vi "PPL RT Driver VI_InlineAsync.vi"(7 "Operation":T1, 11 "Device Reference in":T2 format="%.0x") -> (0 "Error Code":i32)   [LabVIEW 2020]
uses:
  <vilib>/NI/NIVS Inline Async API/_VS Inline Async API/VS Inline Async API/VS Inline Async API.lvclass
  <vilib>/NI VeriStand/Custom Device API/Custom Device API.lvlib
  <vilib>/NI VeriStand/Custom Device Tools/Custom Device Utility Library/Custom Device Utility Library.lvlib
  <vilib>/NI VeriStand/Custom Device API/Get Item Property (Variant).vi
  <vilib>/NI VeriStand/Custom Device API/Data Reference.ctl
  <vilib>/NI VeriStand/Custom Device API/Block Data Reference.ctl
  <vilib>/NI VeriStand/Custom Device API/Custom Device Item Ref.ctl
  <vilib>/NI VeriStand/Custom Device API/Hardware Interface Driver VI Operation.ctl
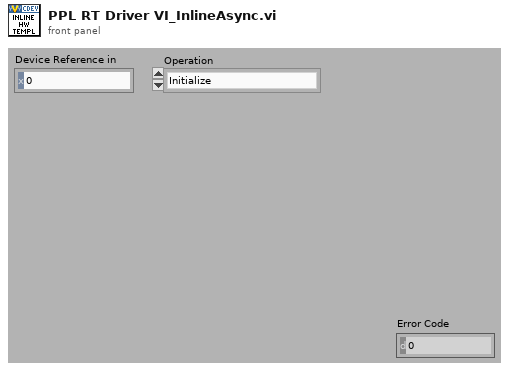
[diagram p1: front panel]
types:
  T1 = typedef "Custom Device API.lvlib/Hardware Interface Driver VI Operation.ctl" = enum16{"Initialize", "Start", "Read Data from HW", "Write Data to HW", "Close"}
  T2 = typedef "Custom Device API.lvlib/Custom Device Item Ref.ctl" = u64
  T3 = cluster{"Async":refnum<class "VS Inline Async API.lvclass">, "Settings":cluster{"Name":string, "Async Init Timeout":u16}}
  T4 = typedef "Custom Device API.lvlib/Block Data Reference.ctl" = cluster{"Data Reference":T5, "Offset":u64, "Length":u64}
  T5 = typedef "Custom Device API.lvlib/Data Reference.ctl" = i32
  T6 = cluster{"Name":string, "Async Init Timeout":u16, "Compiled.InlineAsync.Settings":cluster{"Read":cluster{"Refs":T4[], "Values":dbl[]}[], "Write":cluster{"Refs":T4[], "Values":dbl[]}[], "ReadWrite":cluster{"Refs":T5[], "Values":dbl[], "Reset Values":dbl[]}[], "LUT":variant}}
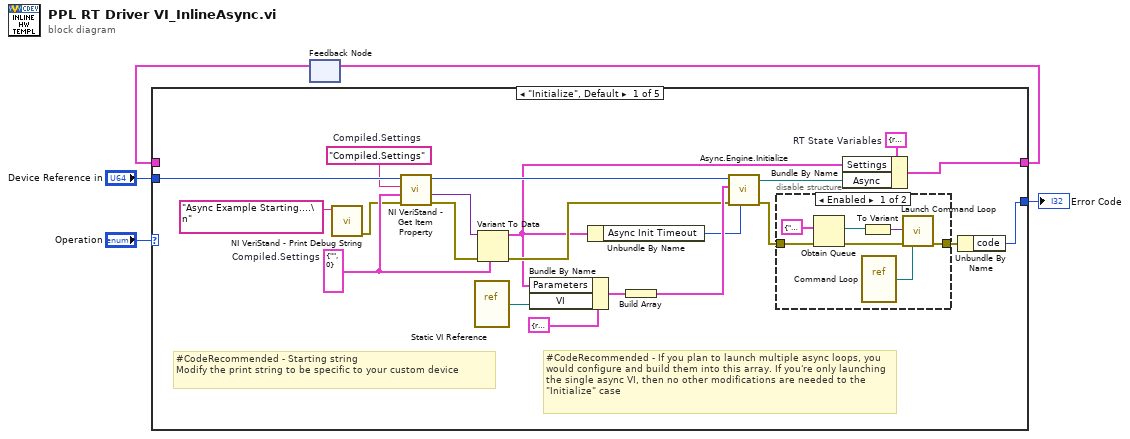
[diagram p0: block diagram]
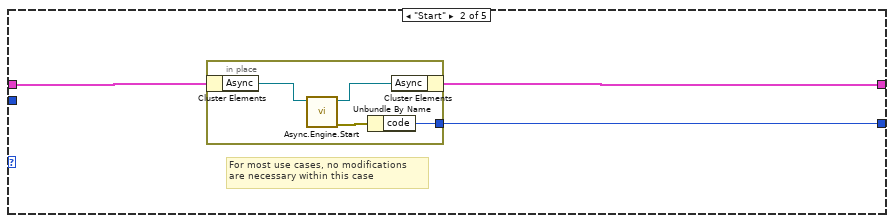
[diagram p3: hidden frame]
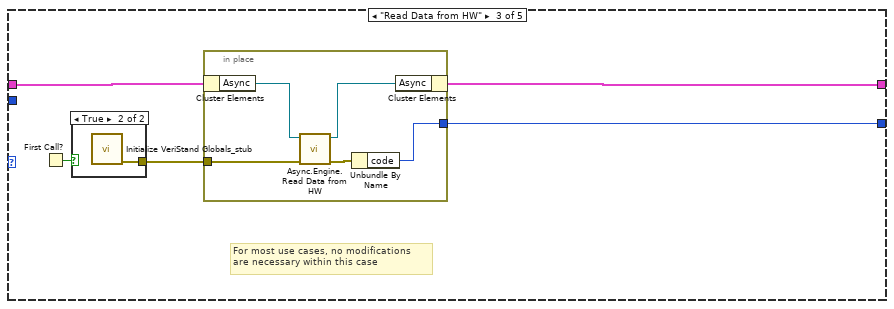
[diagram p4: hidden frame]
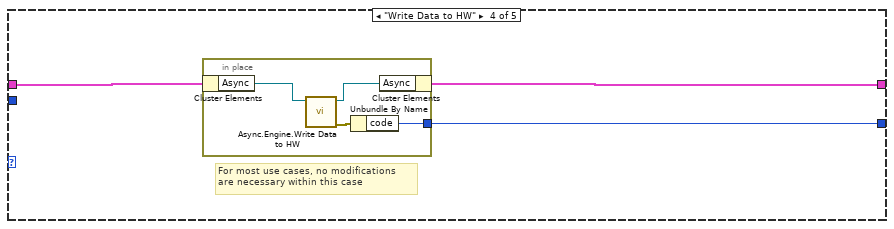
[diagram p6: hidden frame]
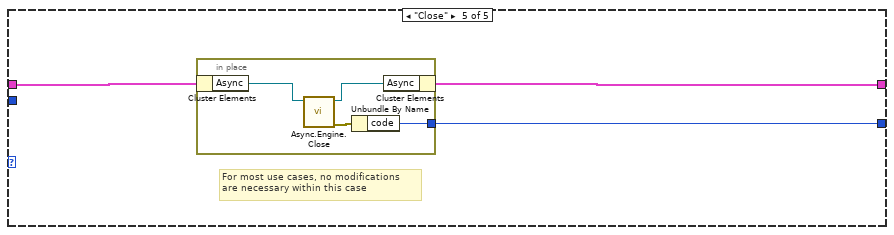
[diagram p7: hidden frame]
diagram:
  n1 = feedback #1() -> (w3:T3)  [unwired: 1 out]
  n2 = case shown="\"Initialize\", Default" "Operation" {
    tunnel: [w24 w36 w44 w53 w61] -> w4
    tunnel: w3 -> [_ w37 w46 w54 w62]
    tunnel: "Device Reference in" -> [w21 _ _ _ _]
    tunnel: [w26 w35 w45 w55 w60] -> w1
    frame "Initialize", Default {
      w16 = T3 {"Async"=refnum, "Settings"={"Name"="", "Async Init Timeout"=0}}  # RT State Variables
      w17 = cluster{"Name":string, "Async Init Timeout":u16} {"Name"="", "Async Init Timeout"=0}  # Compiled.Settings
      w18 = "Compiled.Settings"  # Compiled.Settings
      # "#CodeRecommended - Starting string\nModify the print string to be specific to your custom device"
      # "#CodeRecommended - If you plan to launch multiple async loops, you would configure and build them into this array. If you're only launching the single async VI, then no other modifications are needed to the \"Initialize\" case"
      n3 = call <vilib>:"NI VeriStand - Print Debug String.vi"("Message"="Async Example Starting....\n") -> ("error out"=w12:errorcluster)  [unwired: 10 in]
      n4 = call-poly <vilib>:"NI VeriStand - Get Item Property.vi"("error in (no error)"=w12, "Default Value"=w17, "Property Name"=w18, "Item Ref in"=w21) -> ("error out"=w20:errorcluster, "Value"=w19:variant, "Item Ref out"=w13:T2)  [unwired: 4 in, 1 out]
      n5 = vi-ref "Static VI Reference"() -> ("vi reference"=w10:refnum<vi>)
      n6 = Variant To Data(error in=w20, type=w17, Variant=w19) -> (data=w9:cluster{"Name":string, "Async Init Timeout":u16}, error out=w14:errorcluster)
      n7 = Bundle By Name(cluster=cluster{"VI":refnum<vi>, "Parameters":variant} {"VI"=refnum, "Parameters"=variant} ("Process"), "Parameters"=w9, "VI"=w10) -> (w22:cluster{"VI":refnum<vi>, "Parameters":variant})
      n8 = Unbundle By Name(w9) -> ("Async Init Timeout"=w8:u16)
      n9 = Build Array(w22) -> (w15:cluster{"VI":refnum<vi>, "Parameters":variant}[])
      n10 = call <vilib>:"Async.Engine.Initialize.vi"("Timeout (ms) (5000)"=w8, "error in (no error)"=w14, "Processes"=w15, "Custom Device Ref"=w13) -> ("error out"=w7:errorcluster, "Async"=w25:refnum<class "VS Inline Async API.lvclass">)  [unwired: 6 in]
      n11 = disable-structure shown="Enabled" {
        disable-tunnel: w7 -> [w29 w34]
        disable-tunnel: [w30 w34] -> w6
        frame Enabled {
          n12 = Obtain Queue(element data type=T6 {"Name"="", "Async Init Timeout"=0, "Compiled.InlineAsync.Settings"={"Read"=[], "Write"=[], "ReadWrite"=[], "LUT"=variant}} ("Reconfigure.Settings.ctl"), error in (no error)=w29) -> (queue out=w33:refnum<queue>, error out=w31:errorcluster)  [unwired: 3 in, 1 out]
          n13 = vi-ref "Command Loop.vi"() -> (w28:refnum<vi>)
          n14 = To Variant(anything=w33) -> (Variant=w32:variant)
          n15 = call "Launch Command Loop.vi"("VI Refnum"=w28, "error in"=w31, "Queue Refs"=w32) -> ("error out"=w30:errorcluster)  [unwired: 8 in]
        }
        frame Disabled {
        }
      }
      n16 = Bundle By Name(cluster=w16, "Settings"=w9, "Async"=w25) -> (w24:T3)
      n17 = Unbundle By Name(w6) -> ("code"=w26:i32)
    }
    frame "Start" {
      # "For most use cases, no modifications \nare necessary within this case"
      n18 = in-place {
        in-place-border: [w38] -> w35
        n19 = in-place-cluster #2(w37) -> ("Async"=w41:refnum<class "VS Inline Async API.lvclass">)
        n20 = call <vilib>:"Async.Engine.Start.vi"("VS Inline Async API in"=w41) -> ("error out"=w39:errorcluster, "VS Inline Async API out"=w40:refnum<class "VS Inline Async API.lvclass">)  [unwired: 9 in]
        n21 = Unbundle By Name(w39) -> ("code"=w38:i32)
        n22 = in-place-cluster #2("Async"=w40) -> (w36:T3)
      }
    }
    frame "Read Data from HW" {
      # "For most use cases, no modifications \nare necessary within this case"
      n23 = First Call?() -> (First Call?: T/F=w42:bool)
      n24 = case shown="True" w42 {
        tunnel: [_ w47] -> w43
        frame False {
        }
        frame True {
          n25 = call "Initialize VeriStand Globals_stub.vi"() -> ("error out"=w47:errorcluster)  [unwired: 11 in]
        }
      }
      n26 = in-place {
        in-place-border: [w50] -> w45
        in-place-border: w43 -> [w48]
        n27 = in-place-cluster #3(w46) -> ("Async"=w52:refnum<class "VS Inline Async API.lvclass">)
        n28 = call <vilib>:"Async.Engine.Read Data from HW.vi"("error in"=w48, "Async in"=w52) -> ("error out"=w49:errorcluster, "Async out"=w51:refnum<class "VS Inline Async API.lvclass">)  [unwired: 8 in]
        n29 = Unbundle By Name(w49) -> ("code"=w50:i32)
        n30 = in-place-cluster #3("Async"=w51) -> (w44:T3)
      }
    }
    frame "Write Data to HW" {
      # "For most use cases, no modifications \nare necessary within this case"
      n31 = in-place {
        in-place-border: [w59] -> w55
        n32 = in-place-cluster #4(w54) -> ("Async"=w57:refnum<class "VS Inline Async API.lvclass">)
        n33 = call <vilib>:"Async.Engine.Write Data to HW.vi"("VS Inline Async API in"=w57) -> ("error out"=w58:errorcluster, "VS Inline Async API out"=w56:refnum<class "VS Inline Async API.lvclass">)  [unwired: 9 in]
        n34 = Unbundle By Name(w58) -> ("code"=w59:i32)
        n35 = in-place-cluster #4("Async"=w56) -> (w53:T3)
      }
    }
    frame "Close" {
      # "For most use cases, no modifications \nare necessary within this case"
      n36 = in-place {
        in-place-border: [w64] -> w60
        n37 = in-place-cluster #5(w62) -> ("Async"=w66:refnum<class "VS Inline Async API.lvclass">)
        n38 = call <vilib>:"Async.Engine.Close.vi"("Async in"=w66) -> ("error out"=w63:errorcluster, "Async out"=w65:refnum<class "VS Inline Async API.lvclass">)  [unwired: 9 in]
        n39 = Unbundle By Name(w63) -> ("code"=w64:i32)
        n40 = in-place-cluster #5("Async"=w65) -> (w61:T3)
      }
    }
  }
  "Error Code" <- w1
  n41 = feedback-in #1(w4) -> ()
